vi "OutPutOff.vi"(8 "error in (no error)":errorcluster) -> (0 "error out":errorcluster {"code" format="%.0x"})   [LabVIEW 2010]
uses:
  NI Modbus.llb/MB Serial Master Query Write Single Register (poly).vi
panel:
  in  "Cancel":bool
  in  "OK":bool
  # "确认关闭输出?"
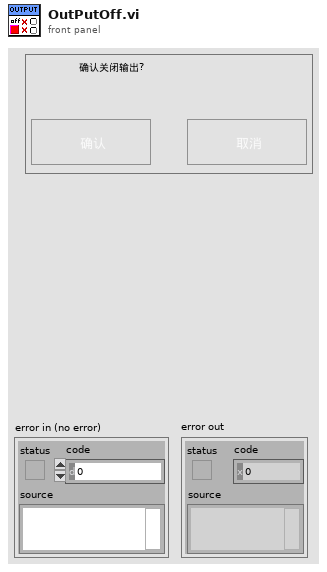
[diagram p1: front panel]
types:
  T1 = cluster{"Mode":enum16{"RTU", "ASCII"}, "Slave Address":u8}
  T2 = typedef "Path InitPaths__FS.ctl" = cluster{"Ctrller CFG":path, "INI":path, "Profile":path, "EventLog":path, "Data":path}
  T3 = typedef "Controller Configuration__CHC.ctl" = cluster{"Ctrller Type":T4, "Ctrller Name":string, "Ctrller Addr":string, "Server IP":string, "Conn Result":string, "Port":string, "Baud":dbl}
  T4 = typedef "Controller Configuration__Ctrller Type.ctl" = enum16{"F4S/D", "Synergy"}
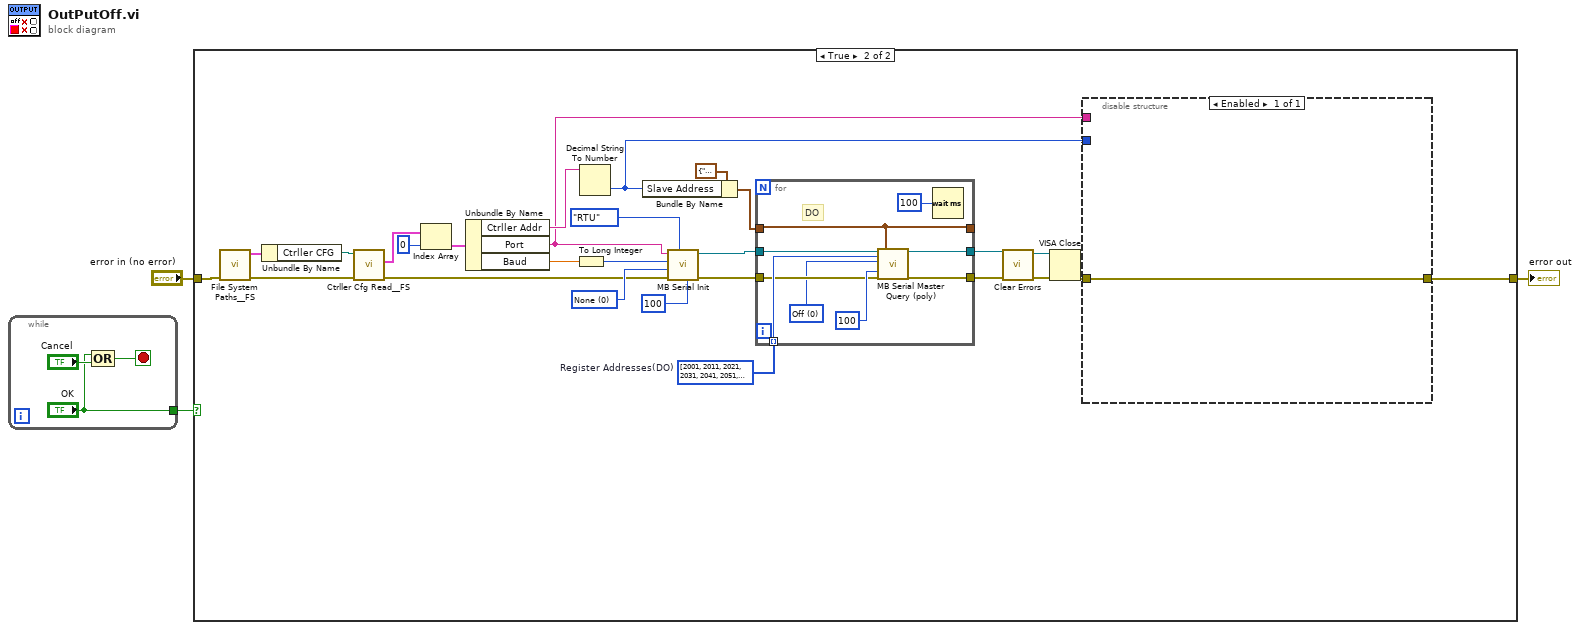
[diagram p0: block diagram]
diagram:
  n1 = while {
    tunnel: ["OK"] -> w3
    stop <- w5 stop-if-true
    n2 = Compound Arithmetic op=OR("OK", "Cancel") -> (w5:bool)
  }
  n3 = case shown="True" w3 {
    tunnel: "error in (no error)" -> [w7 w9]
    tunnel: [w7 w8] -> w1
    frame False {
    }
    frame True {
      w13 = i32[] [2001, 2011, 2021, 2031, 2041, 2051, 2061, 2071]  # Register Addresses(DO)
      w21 = u16 0 items=["None", "Odd", "Even", "Mark", "Space"] ("Parity")
      n4 = call "File System Paths__FS.vi"("error in (no error)"=w9) -> ("error out"=w24:errorcluster, "FilePaths"=w30:T2)  [unwired: 8 in, 1 out]
      n5 = Unbundle By Name(w30) -> ("Ctrller CFG"=w31:path)
      n6 = call "Ctrller Cfg Read__FS.vi"("error in (no error)"=w24, "Path In"=w31) -> ("error out"=w18:errorcluster, "Ctrllers"=w29:T3[])  [unwired: 7 in, 1 out]
      n7 = Index Array(array=w29, index=0) -> (element=w27:T3)
      n8 = Unbundle By Name(w27) -> ("Ctrller Addr"=w26:string, "Port"=w10:string, "Baud"=w25:dbl)
      n9 = To Long Integer(number=w25) -> (32bit integer=w22:i32)
      n10 = Decimal String To Number(string=w26) -> (number=w11:i32)  [unwired: 2 in, 1 out]
      n11 = Bundle By Name(cluster=T1 {"Mode"=enum."RTU", "Slave Address"=0} ("Serial Parameters"), "Slave Address"=w11) -> (w19:T1)
      n12 = call "MB Serial Init.vi"("Timeout"=u32 100, "Mode"=enum16{"RTU", "ASCII"}."RTU", "error in (no error)"=w18, "Parity"=w21, "Baud Rate"=w22, "VISA resource name"=w10) -> ("error out"=w32:errorcluster, "VISA resource name out"=w33:refnum<visa-resource-name>)  [unwired: 4 in]
      n13 = for {
        tunnel: w13 -> [w43] mode=indexing
        tunnel: w33 -> [w42]
        tunnel: w32 -> [w39]
        tunnel: [w38] -> w17
        tunnel: [w37] -> w16
        tunnel: w19 -> [w35]
        tunnel: [w35] -> _
        w36 = u16 0 items=["Off", "Event Output", "Complementary Output", "Control Output / Boost Heat", "Boost Cool", "Compressor"] ("Function (0: Off)")
        # "DO"
        n14 = call-poly "MB Serial Master Query (poly).vi"("VISA resource name"=w42, "Address"=w43, "Holding Register"=w36, "Timeout"=u32 100, "error in"=w39, "Serial Parameters"=w35) -> ("VISA resource name out"=w37:refnum<visa-resource-name>, "error out"=w38:errorcluster)  [unwired: 11 in, 1 out]
        n15 = Wait (ms)(milliseconds to wait=u32 100) -> ()  [unwired: 1 out]
      }
      n16 = call <vilib>:"Clear Errors.vi"("error in (no error)"=w17) -> ("error out"=w15:errorcluster)  [unwired: 6 in]
      n17 = VISA Close(VISA resource name=w16, error in (no error)=w15) -> (error out=w12:errorcluster)
      n18 = disable-structure shown="Enabled" {
        disable-tunnel: w12 -> [w34]
        disable-tunnel: w11 -> [_]
        disable-tunnel: w10 -> [_]
        disable-tunnel: [w34] -> w8
        frame Enabled {
        }
      }
    }
  }
  "error out" <- w1
